vi "Version 1_Write Output Definitions.vi"(6 "Software Version (Optional - wire for speed)":u8, 7 "Address (A)":string="A", 8 "error in":errorcluster, 9 "Read-Only Options (NOT USED, Contact Alicat if these features\nwere needed in your old programs; hardware changes are required\nfor many of these alterations)":T1, 10 "Read/Write Options":T2, 11 "VISA Session In":refnum<visa-resource-name>="Alicat") -> (0 "error out":errorcluster, 3 "VISA Session Out":refnum<visa-resource-name>)   [LabVIEW 2015]
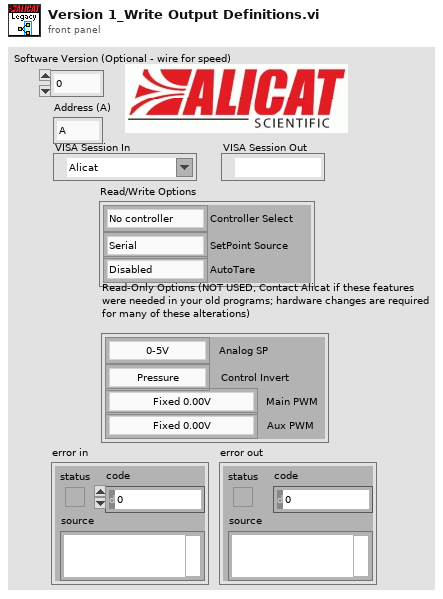
[diagram p1: front panel]
types:
  T1 = cluster{"Analog SP":enum16{"0-5V", "4-20mA"}, "Control Invert":enum16{"Pressure", "Vacuum/BP"}, "Main PWM":enum8{"Fixed 0.00V", "Pressure 0-5V", "Temperature 0-5V", "Volumetric Flow 0-5V", "Mass Flow 0-5V", "Pressure 0-2.5-5V bidir", "Temperature 0-2.5-5V bidir", "Volumetric Flow 0-2.5-5V bidir", "Mass Flow 0-2.5-5V bidir", "Pressure 1-5V", "Temperature 1-5V", "Volumetric Flow 1-5V", "Mass Flow 1-5V", "Reserved(A)", "Reserved(B)", "Fixed 5.12V"}, "Aux PWM":enum8{"Fixed 0.00V", "Pressure 0-5V", "Temperature 0-5V", "Volumetric Flow 0-5V", "Mass Flow 0-5V", "Pressure 0-2.5-5V bidir", "Temperature 0-2.5-5V bidir", "Volumetric Flow 0-2.5-5V bidir", "Mass Flow 0-2.5-5V bidir", "Pressure 1-5V", "Temperature 1-5V", "Volumetric Flow 1-5V", "Mass Flow 1-5V", "Reserved(A)", "Reserved(B)", "Fixed 5.12V"}}
  T2 = cluster{"Controller Select":enum8{"No controller", "Pressure", "Temperature", "Volumetric Flow", "Mass Flow", "Unknown"}, "SetPoint Source":enum8{"Serial", "Local", "Analog", "Unknown"}, "AutoTare":enum16{"Disabled", "Enabled"}}
  T3 = cluster{"Controller Select":u16, "SetPoint Source":enum8{"Serial", "Local", "Analog", "Unknown"}, "AutoTare":enum16{"Disabled", "Enabled"}}
  T4 = enum8{"No controller", "Pressure", "Temperature", "Volumetric Flow", "Mass Flow", "Unknown"}
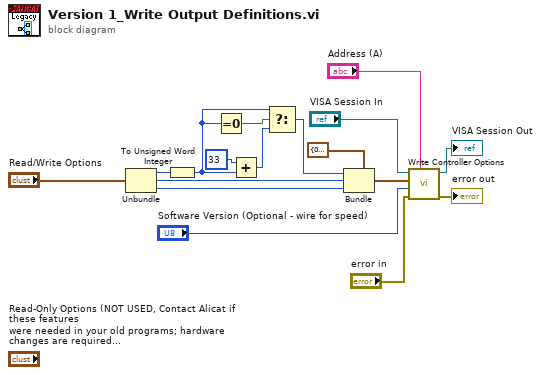
[diagram p0: block diagram]
diagram:
  n1 = Unbundle("Read/Write Options") -> ("Controller Select"=w6:T4, "SetPoint Source"=w8:enum8{"Serial", "Local", "Analog", "Unknown"}, "AutoTare"=w7:enum16{"Disabled", "Enabled"})
  n2 = To Unsigned Word Integer(number=w6) -> (unsigned 16bit integer=w3:u16)
  n3 = Equal To 0?(x=w3) -> (x = 0?=w4:bool)
  n4 = Add(x=u16 33, y=w3) -> (x+y=w2:u16)
  n5 = Select(t=w3, s=w4, f=w2) -> (s? t:f=w1:u16)
  n6 = Bundle(cluster=T3 {"Controller Select"=0, "SetPoint Source"=enum."Serial", "AutoTare"=enum."Disabled"} ("Read/Write Options"), "Controller Select"=w1, "SetPoint Source"=w8, "AutoTare"=w7) -> (w10:T3)
  n7 = call "Write Controller Options.vi"("Unit ID (A)"="Address (A)", "error in"="error in", "Software Version"="Software Version (Optional - wire for speed)", "Read/Write Options"=w10, "VISA Session In"="VISA Session In") -> ("error out"=→"error out":errorcluster, "VISA Session Out"=→"VISA Session Out":refnum<visa-resource-name>)  [unwired: 5 in]
